vi "Start Print.vi"(8 "error in (no error)":errorcluster, 11 "Feeder Actor.lvlib:Mixer.lvclass":refnum<class "Mixer.lvclass">) -> (0 "error out":errorcluster, 3 "Feeder Actor.lvlib:Mixer.lvclass 2":refnum<class "Mixer.lvclass">)   [LabVIEW 2018, in "Feeder Actor.lvlib" / "Mixer.lvclass"]
uses:
  Mixer.lvclass
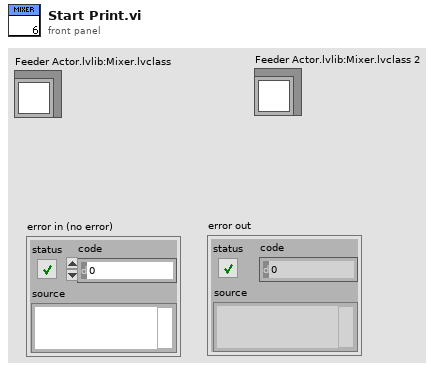
[diagram p1: front panel]
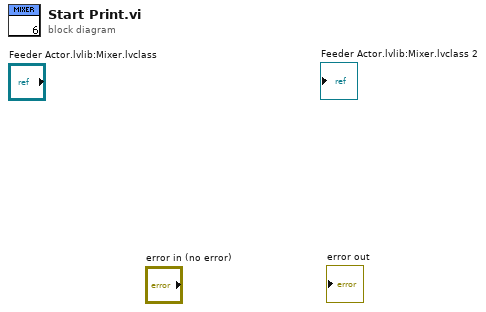
[diagram p0: block diagram]
diagram:
